vi "ArmStates.vi"(9 "Mode":string="Carry") -> ()   [LabVIEW 2020]
uses:
  <vilib>/Rock Robotics/WPI/ThirdParty/REV Robotics/REVLib/Typedef/Spark MAX Control Type.ctl
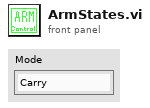
[diagram p1: front panel]
types:
  T1 = typedef "Spark MAX Control Type.ctl" = enum16{"Percent VBus", "Voltage", "Velocity", "Position", "Smart Motion", "Current", "Smart Velocity"}
  T2 = typedef "WPI_MotorControlDeviceRef.ctl" = cluster{"DeviceStatus":errorcluster, "Type":T3, "PWM":cluster{"PWM Channel":T4, "DeadBand":T5}, "CAN":cluster{"Device Number":u8, "SetOutput VI Ref":variant, "GetOutput VI Ref":variant, "Enable VI Ref":variant, "Disable VI Ref":variant, "Data":variant}, "Invert":bool, "DIO PWM":cluster{"PWM \"Enable\" Channel":T4, "DIOChannel":T6, "PWM Rate":dbl}}
  T3 = typedef "WPI_MotorControlType.ctl" = enum16{"PWM", "CAN", "DIO PWM"}
  T4 = typedef "FPGA_DIOPWMChannel.ctl" = enum8{"PWM 0", "PWM 1", "PWM 2", "PWM 3", "PWM 4", "PWM 5", "PWM 6", "PWM 7", "PWM 8", "PWM 9", "PWM MXP 0", "PWM MXP 1", "PWM MXP 2", "PWM MXP 3", "PWM MXP 4", "PWM MXP 5", "PWM MXP 6", "PWM MXP 7", "PWM MXP 8", "PWM MXP 9", "Invalid"}
  T5 = typedef "WPI_PWMDeadband.ctl" = cluster{"Name":string, "maxPositivePwm":i32, "minPositivePwm":i32, "centerPwm":i32, "maxNegativePwm":i32, "minNegativePwm":i32, "angularRange":u16}
  T6 = typedef "FPGA_DIOChannel.ctl" = enum8{"DIO 0", "DIO 1", "DIO 2", "DIO 3", "DIO 4", "DIO 5", "DIO 6", "DIO 7", "DIO 8", "DIO 9", "DIO MXP 0", "DIO MXP 1", "DIO MXP 2", "DIO MXP 3", "DIO MXP 4", "DIO MXP 5", "DIO MXP 6", "DIO MXP 7", "DIO MXP 8", "DIO MXP 9", "DIO MXP 10", "DIO MXP 11", "DIO MXP 12", "DIO MXP 13", "DIO MXP 14", "DIO MXP 15", "SPI Port CS1", "SPI Port CS2", "SPI Port CS3", "SPI Port MISO", "SPI Port MOSI", "Invalid"}
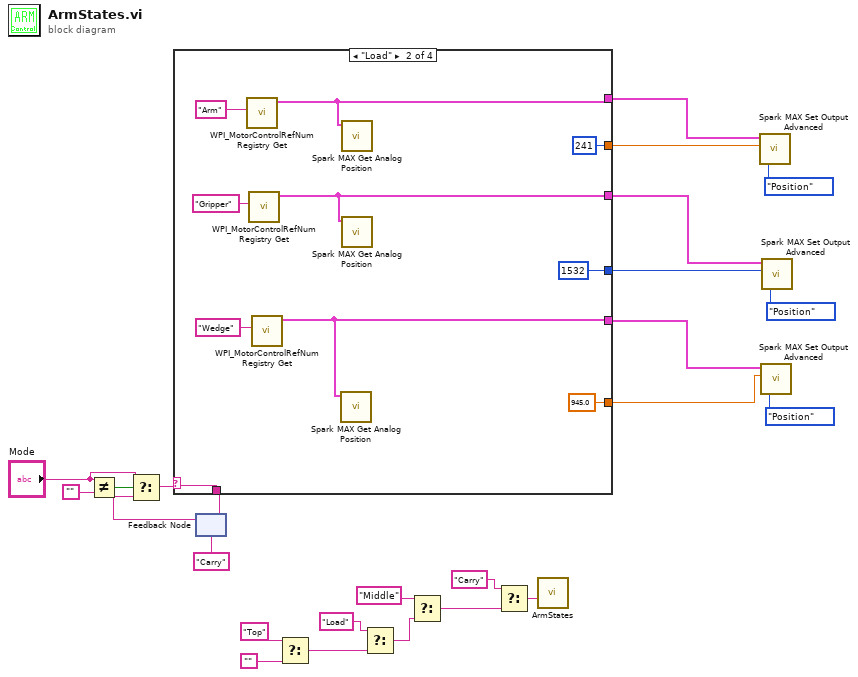
[diagram p0: block diagram]
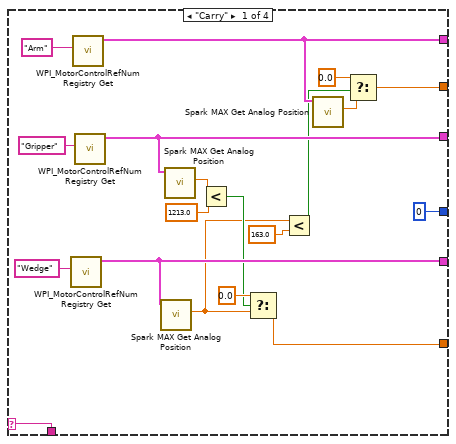
[diagram p2: hidden frame]
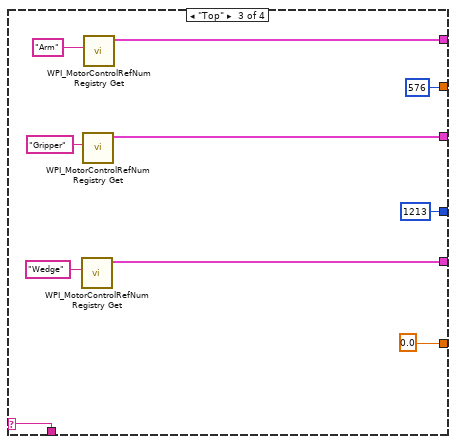
[diagram p3: hidden frame]
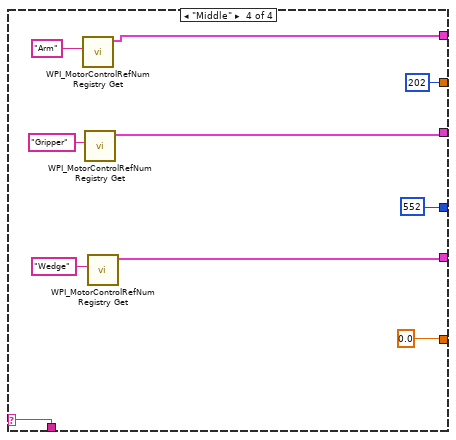
[diagram p4: hidden frame]
diagram:
  n1 = Not Equal?(x="Mode", y="") -> (x != y?=w22:bool)
  n2 = feedback #1("Carry") -> (w24:string)
  n3 = Select(t="Mode", s=w22, f=w24) -> (s? t:f=w25:string)
  n4 = case shown="\"Load\"" w25 {
    selector: w25 -> [w48 w58 w68 w76]
    tunnel: [w48 w58 w68 w76] -> w23
    tunnel: [0 1532 1213 552] -> w20
    tunnel: [w40 241 576 202] -> w19
    tunnel: [w31 945.0 ("f") 0.0 ("f") 0.0 ("f")] -> w17
    tunnel: [w39 w52 w61 w71] -> w16
    tunnel: [w44 w51 w60 w70] -> w15
    tunnel: [w36 w50 w59 w69] -> w14
    frame "Carry" {
      n5 = call <vilib>:"WPI_MotorControlRefNum Registry Get.vi"("refnum name"="Wedge") -> ("MotorControlDevRef"=w36:T2)  [unwired: 9 in, 1 out]
      n6 = call <vilib>:"WPI_MotorControlRefNum Registry Get.vi"("refnum name"="Arm") -> ("MotorControlDevRef"=w39:T2)  [unwired: 9 in, 1 out]
      n7 = call <vilib>:"WPI_MotorControlRefNum Registry Get.vi"("refnum name"="Gripper") -> ("MotorControlDevRef"=w44:T2)  [unwired: 9 in, 1 out]
      n8 = call <vilib>:"Spark MAX Get Analog Position.vi"("MotorControlDevRef in"=w36) -> ("Analog Position"=w30:dbl)  [unwired: 7 in, 3 out]
      n9 = call <vilib>:"Spark MAX Get Analog Position.vi"("MotorControlDevRef in"=w44) -> ("Analog Position"=w43:dbl)  [unwired: 7 in, 3 out]
      n10 = Less?(x=w43, y=1213.0) -> (x < y?=w34:bool)
      n11 = Select(t=0.0, s=w34, f=w30) -> (s? t:f=w31:dbl)
      n12 = Less?(x=w30, y=163.0) -> (x < y?=w32:bool)
      n13 = call <vilib>:"Spark MAX Get Analog Position.vi"("MotorControlDevRef in"=w39) -> ("Analog Position"=w38:dbl)  [unwired: 7 in, 3 out]
      n14 = Select(t=0.0, s=w32, f=w38) -> (s? t:f=w40:dbl)
    }
    frame "Load" {
      n15 = call <vilib>:"WPI_MotorControlRefNum Registry Get.vi"("refnum name"="Arm") -> ("MotorControlDevRef"=w52:T2)  [unwired: 9 in, 1 out]
      n16 = call <vilib>:"WPI_MotorControlRefNum Registry Get.vi"("refnum name"="Gripper") -> ("MotorControlDevRef"=w51:T2)  [unwired: 9 in, 1 out]
      n17 = call <vilib>:"WPI_MotorControlRefNum Registry Get.vi"("refnum name"="Wedge") -> ("MotorControlDevRef"=w50:T2)  [unwired: 9 in, 1 out]
      n18 = call <vilib>:"Spark MAX Get Analog Position.vi"("MotorControlDevRef in"=w50) -> ()  [unwired: 7 in, 4 out]
      n19 = call <vilib>:"Spark MAX Get Analog Position.vi"("MotorControlDevRef in"=w52) -> ()  [unwired: 7 in, 4 out]
      n20 = call <vilib>:"Spark MAX Get Analog Position.vi"("MotorControlDevRef in"=w51) -> ()  [unwired: 7 in, 4 out]
    }
    frame "Top" {
      n21 = call <vilib>:"WPI_MotorControlRefNum Registry Get.vi"("refnum name"="Wedge") -> ("MotorControlDevRef"=w59:T2)  [unwired: 9 in, 1 out]
      n22 = call <vilib>:"WPI_MotorControlRefNum Registry Get.vi"("refnum name"="Gripper") -> ("MotorControlDevRef"=w60:T2)  [unwired: 9 in, 1 out]
      n23 = call <vilib>:"WPI_MotorControlRefNum Registry Get.vi"("refnum name"="Arm") -> ("MotorControlDevRef"=w61:T2)  [unwired: 9 in, 1 out]
    }
    frame "Middle" {
      n24 = call <vilib>:"WPI_MotorControlRefNum Registry Get.vi"("refnum name"="Arm") -> ("MotorControlDevRef"=w71:T2)  [unwired: 9 in, 1 out]
      n25 = call <vilib>:"WPI_MotorControlRefNum Registry Get.vi"("refnum name"="Gripper") -> ("MotorControlDevRef"=w70:T2)  [unwired: 9 in, 1 out]
      n26 = call <vilib>:"WPI_MotorControlRefNum Registry Get.vi"("refnum name"="Wedge") -> ("MotorControlDevRef"=w69:T2)  [unwired: 9 in, 1 out]
    }
  }
  n27 = feedback-in #1(w23) -> ()
  n28 = Select(t="Top", f="") -> (s=w9:bool, s? t:f=w7:string)
  n29 = Select(t="Load", f=w7) -> (s=w10:bool, s? t:f=w11:string)
  n30 = Select(t="Middle", f=w11) -> (s=w1:bool, s? t:f=w12:string)
  n31 = Select(t="Carry", f=w12) -> (s=w13:bool, s? t:f=w3:string)
  n32 = call "ArmStates.vi"("Mode"=w3) -> ()  [unwired: 11 in]
  n33 = call <vilib>:"Spark MAX Set Output Advanced.vi"("Control Mode"=Spark_MAX_Control_Type."Position", "Setpoint"=w19, "MotorControlDevRef"=w16) -> ()  [unwired: 7 in, 2 out]
  n34 = call <vilib>:"Spark MAX Set Output Advanced.vi"("Control Mode"=Spark_MAX_Control_Type."Position", "Setpoint"=w17, "MotorControlDevRef"=w14) -> ()  [unwired: 7 in, 2 out]
  n35 = call <vilib>:"Spark MAX Set Output Advanced.vi"("Control Mode"=Spark_MAX_Control_Type."Position", "Setpoint"=w20, "MotorControlDevRef"=w15) -> ()  [unwired: 7 in, 2 out]
